vi "Updata Cards by DevsInfo.vi"(8 "error in (no error)":errorcluster caption="错误输入（无错误）", 10 "DevsInfo":T1[](array[typedef]), 11 "Cards in":T1[](array[typedef])) -> (0 "error out":errorcluster caption="错误输出", 3 "Cards out":T1[](array[typedef]))   [LabVIEW 2016]
uses:
  Controls/PSCHN_Card Para.ctl
  Controls/PSCHN_Channel Para.ctl
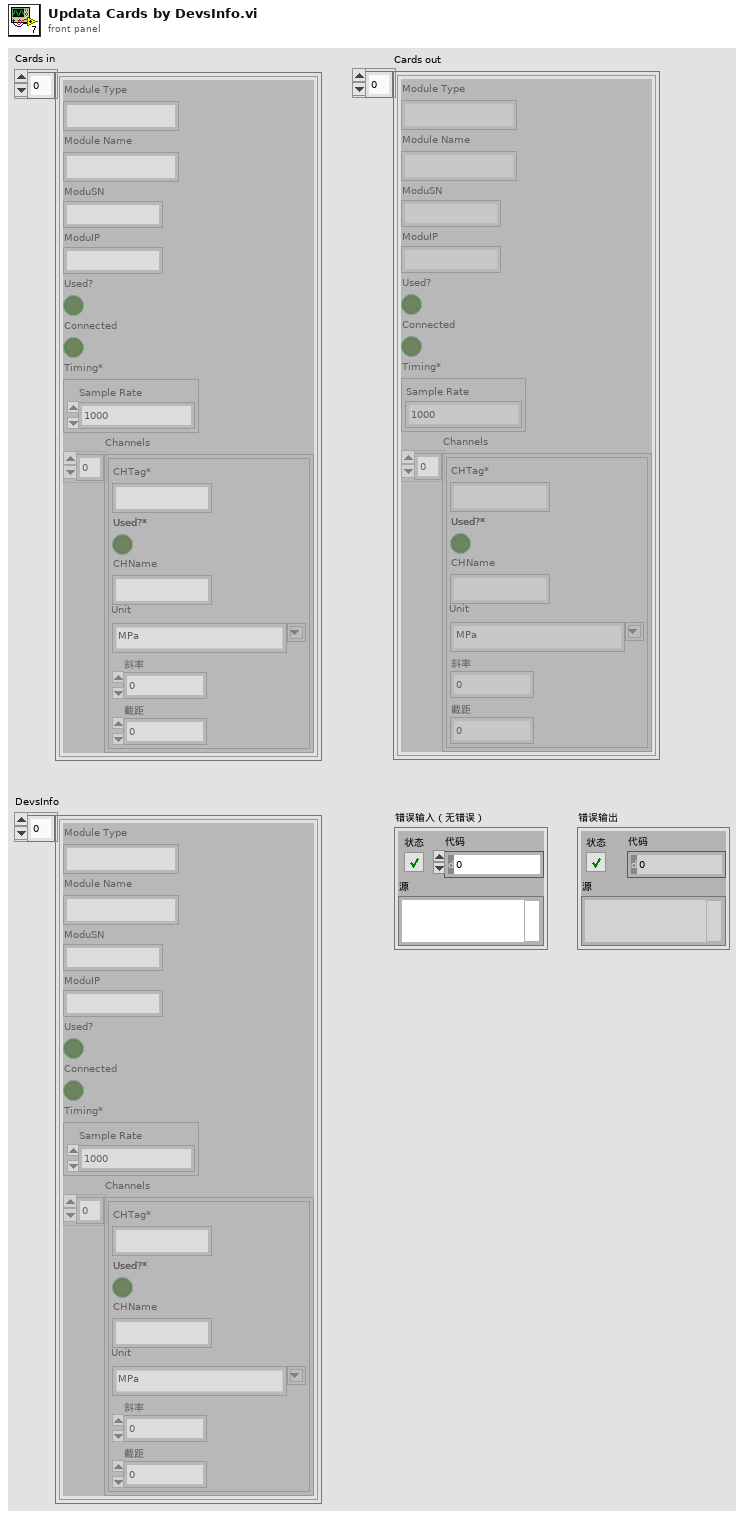
[diagram p1: front panel]
types:
  T1 = typedef "PSCHN_Card Para.ctl" = cluster{"Module Type":string, "Module Name":string, "ModuSN":string, "ModuIP":string, "Used?":bool, "Connected":bool, "Timing*":cluster{"Sample Rate":dbl}, "Channels":T2[]}
  T2 = typedef "PSCHN_Channel Para.ctl" = cluster{"CHTag*":string, "Used?*":bool, "CHName":string, "Unit":string, "斜率":dbl, "截距":dbl}
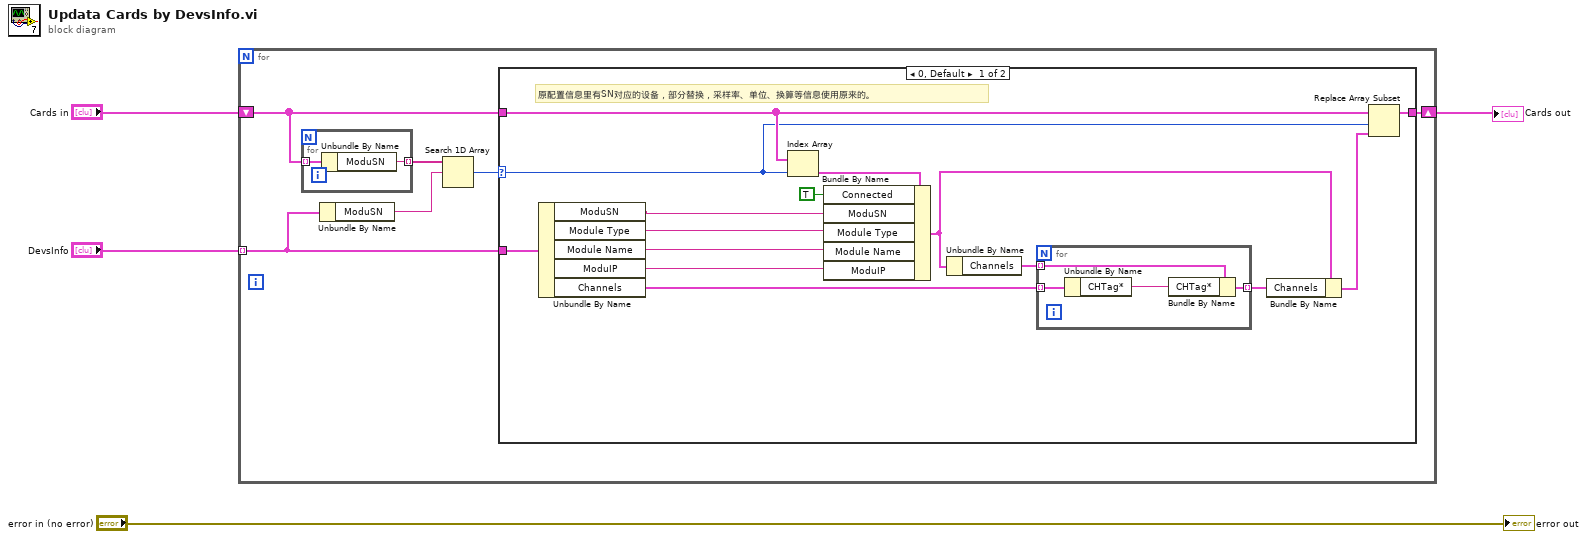
[diagram p0: block diagram]
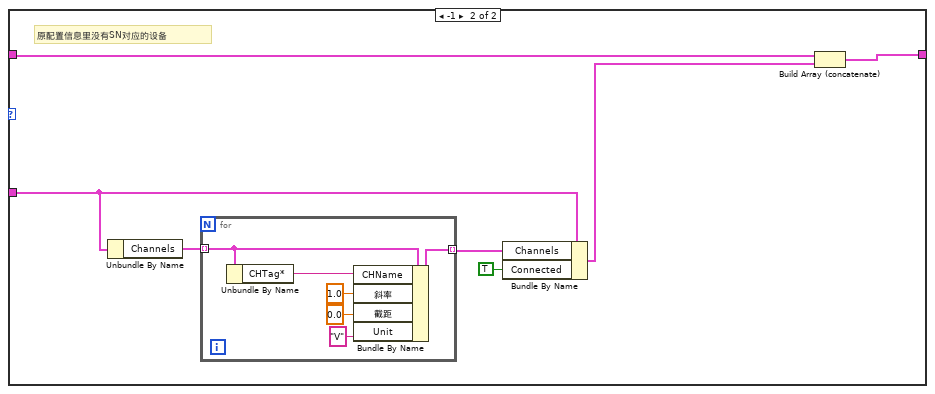
[diagram p2: hidden frame]
diagram:
  n1 = for {
    tunnel: "DevsInfo" -> [w5] mode=indexing
    shift-right: [w7] -> w1
    shift-left: "Cards in" -> [w9]
    n2 = for {
      tunnel: w9 -> [w44] mode=indexing
      tunnel: [w43] -> w10 mode=indexing
      n3 = Unbundle By Name(w44) -> ("ModuSN"=w43:string)
    }
    n4 = Unbundle By Name(w5) -> ("ModuSN"=w8:string)
    n5 = Search 1D Array(1D array=w10, element=w8) -> (index of element=w6:i32)  [unwired: 1 in]
    n6 = case shown="0, Default" w6 {
      selector: w6 -> [w18 _]
      tunnel: w9 -> [w25 w32]
      tunnel: [w19 w30] -> w7
      tunnel: w5 -> [w16 w33]
      frame 0, Default {
        # "原配置信息里有SN对应的设备，部分替换，采样率、单位、换算等信息使用原来的。"
        n7 = Unbundle By Name(w16) -> ("ModuSN"=w15:string, "Module Type"=w14:string, "Module Name"=w13:string, "ModuIP"=w12:string, "Channels"=w11:T2[])
        n8 = Index Array(array=w25, index=w18) -> (element=w24:T1)
        n9 = Bundle By Name(cluster=w24, "Connected"=TRUE, "ModuSN"=w15, "Module Type"=w14, "Module Name"=w13, "ModuIP"=w12) -> (w21:T1)
        n10 = Unbundle By Name(w21) -> ("Channels"=w23:T2[])
        n11 = for {
          tunnel: w23 -> [w29] mode=indexing
          tunnel: [w27] -> w22 mode=indexing
          tunnel: w11 -> [w26] mode=indexing
          n12 = Unbundle By Name(w26) -> ("CHTag*"=w28:string)
          n13 = Bundle By Name(cluster=w29, "CHTag*"=w28) -> (w27:T2)
        }
        n14 = Bundle By Name(cluster=w21, "Channels"=w22) -> (w20:T1)
        n15 = Replace Array Subset(array=w25, new element=w20, index=w18) -> (w19:T1[])
      }
      frame -1 {
        # "原配置信息里没有SN对应的设备"
        n16 = Unbundle By Name(w33) -> ("Channels"=w36:T2[])
        n17 = for {
          tunnel: w36 -> [w39] mode=indexing
          tunnel: [w40] -> w34 mode=indexing
          n18 = Unbundle By Name(w39) -> ("CHTag*"=w38:string)
          n19 = Bundle By Name(cluster=w39, "CHName"=w38, "斜率"=1.0, "截距"=0.0, "Unit"="V") -> (w40:T2)
        }
        n20 = Bundle By Name(cluster=w33, "Channels"=w34, "Connected"=TRUE) -> (w31:T1)
        n21 = Build Array (concatenate)(w32, w31) -> (w30:T1[])
      }
    }
  }
  "Cards out" <- w1
  "error out" <- "error in (no error)"
